vi "Auto.vi"() -> ()   [LabVIEW 2020]
uses:
  Global_Variable/A180648.vi
  Global_Variable/Global.vi
  Libraries/S7/S7.lvlib
  <userlib>/_MGI/1D Array/MGI Running Average/MGI Running Average(DBL[]).vi
panel:
  out "标尺_Event":refnum<user-event>
  in  "STEP":string
  in  "更换坐标":refnum<vi>
  out "试验项_Event":refnum<user-event>
  out "NVH":bool=TRUE
  out "T1+T2":dbl
  out "T2":dbl
  out "T1":dbl
  out "吸收电流":sgl
  out "输出扭矩(大)":sgl
  out "输入扭矩":sgl
  out "力特性逆向去程":bool
  out "力特性正向去程":bool
  out "力特性逆向回程":bool
  out "力特性正向回程":bool
  out "逆向空载正向初始化":bool
  out "锁紧/开启初始化":bool
  out "功能正向初始化":bool
  out "功能逆向初始化":bool
  out "空载逆向初始化":bool
  out "空载正向初始化":bool
  out "当前车速":i32
  out "试验项目":T1(tab)
  out "手柄锁紧力试验":cluster{dbl[], dbl[]}[](graph)
  out "手柄开启力试验":cluster{dbl[], dbl[]}[](graph)
  out "角度调节力试验":cluster{dbl[], dbl[]}[](graph)
  out "管柱保持力试验":cluster{dbl[], dbl[]}[](graph)
  out "锁紧/开启":cluster{dbl[], dbl[]}[](graph)
  out "逆向空载试验":cluster{dbl[], dbl[]}[](graph)
  out "振动2NHV-FFT":cluster{"f0":dbl, "df":dbl, "magnitude":dbl[]}[](graph)
  out "振动1NVH-FFT":cluster{"f0":dbl, "df":dbl, "magnitude":dbl[]}[](graph)
  in  "判定结果":bool[][](array[boolean])=[[TRUE]]
  # "."
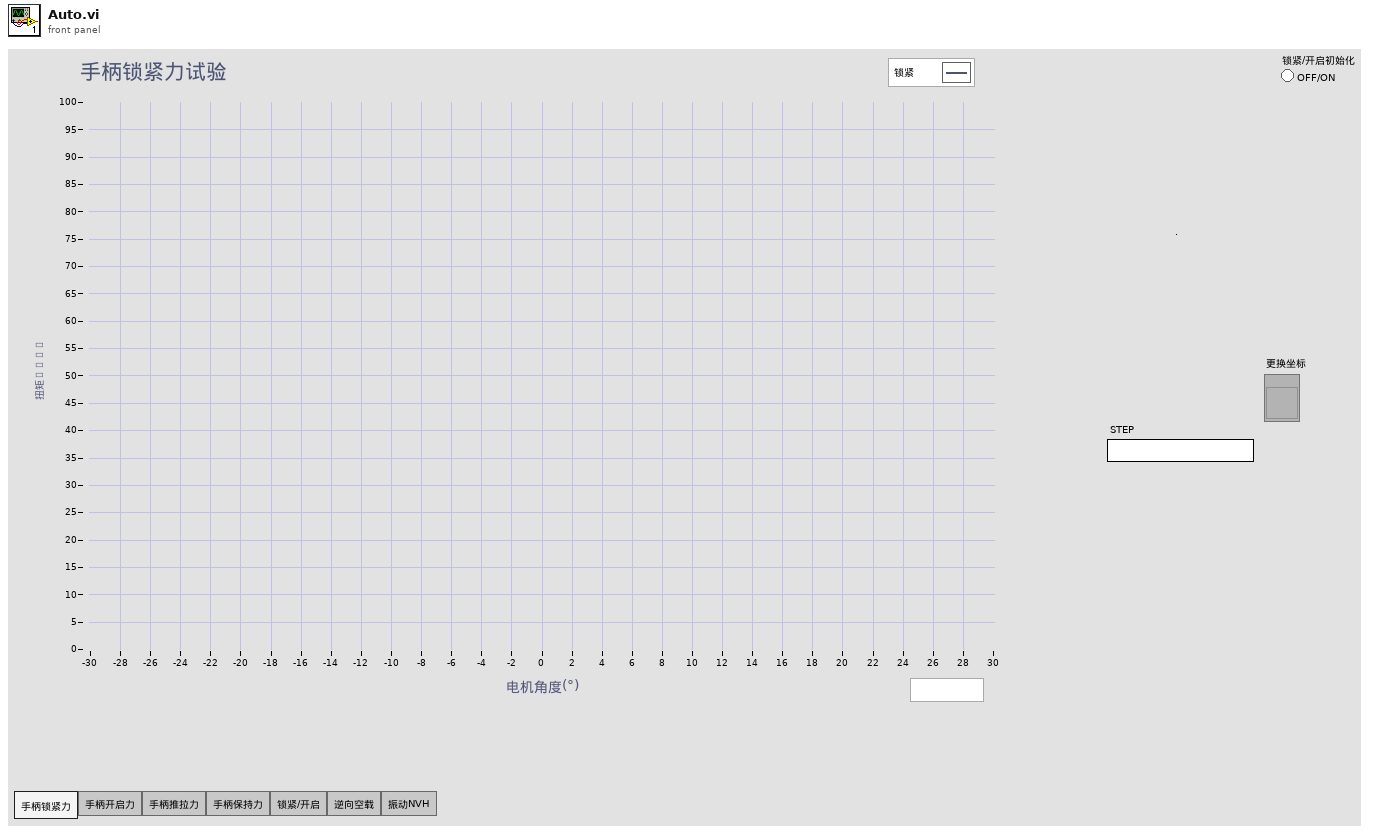
[diagram p1: front panel]
types:
  T1 = enum32{"手柄锁紧力", "手柄开启力", "手柄推拉力", "手柄保持力", "锁紧/开启", "逆向空载", "振动NVH"}
  T2 = enum32{"Invalid", "Standard", "Closed", "Hidden", "Minimized", "Maximized"}
  T3 = enum32{"手柄锁紧力", "手柄开启力", "手柄推拉力", "手柄保持力", "锁紧/开启", "逆向空载", "振动NVH", "完成"}
  T4 = cluster{"输入轴扭矩":dbl, "输出轴扭矩小量程":dbl, "输出轴扭矩大量程":dbl}
  T5 = cluster{"锁紧判断范围":cluster{"单位":string, "下限":dbl, "上限":dbl}}
  T6 = cluster{"开启判断范围":cluster{"单位":string, "下限":dbl, "上限":dbl}}
  T7 = cluster{"推拉力判断范围 ":cluster{"单位":string, "下限":dbl, "上限":dbl}}
  T8 = cluster{"保持力判断范围 ":cluster{"单位":string, "下限":dbl, "上限":dbl}, "保持力监控位移":cluster{"单位":string, "下限":dbl, "上限":dbl}}
  T9 = typedef "lveventtype.ctl" = enum32{"Null", "Timeout", "Annotation Menu Selection", "Annotation Menu Selection?", "App Instance Close", "App Instance Close?", "Autoscale Range Change", "Bookmark Info Change", "Cell Edit", "Cell Edit?", "Cursor Grab", "Cursor Grab?", "Cursor Menu Selection", "Cursor Menu Selection?", "Cursor Move", "Cursor Release", "Data Change", "Direction Change", "Display State Change", "Drag Ended", "Drag Enter", "Drag Leave", "Drag Over", "Drag Source Update", "Drag Starting", "Drag Starting?", "Drop", "Exec State Change", "Key Down", "Key Down?", "Key Repeat", "Key Repeat?", "Key Up", "Listbox Double Click", "Menu Activation?", "Menu Selection (App)", "Menu Selection? (App)", "Menu Selection (User)", "Mouse Down", "Mouse Down?", "Mouse Enter", "Mouse Leave", "Mouse Move", "Mouse Up", "Mouse Wheel", "NI Security User Change (App)", "Pane Size", "Panel Close", "Panel Close?", "Panel Resize", "Plot Attribute Change", "Scale Range Change", "Shortcut Menu Activation?", "Shortcut Menu Selection (App)", "Shortcut Menu Selection? (App)", "Shortcut Menu Selection (User)", "Tree Double Click", "Tree Drag", "Tree Drag?", "Tree Drop", "Tree Drop?", "Tree Item Close", "Tree Item Close?", "Tree Item Open", "Tree Item Open?", "User Event", "Value Change"}
  T10 = typedef "LVPoint32TypeDef.ctl" = cluster{"Horizontal":i32, "Vertical":i32}
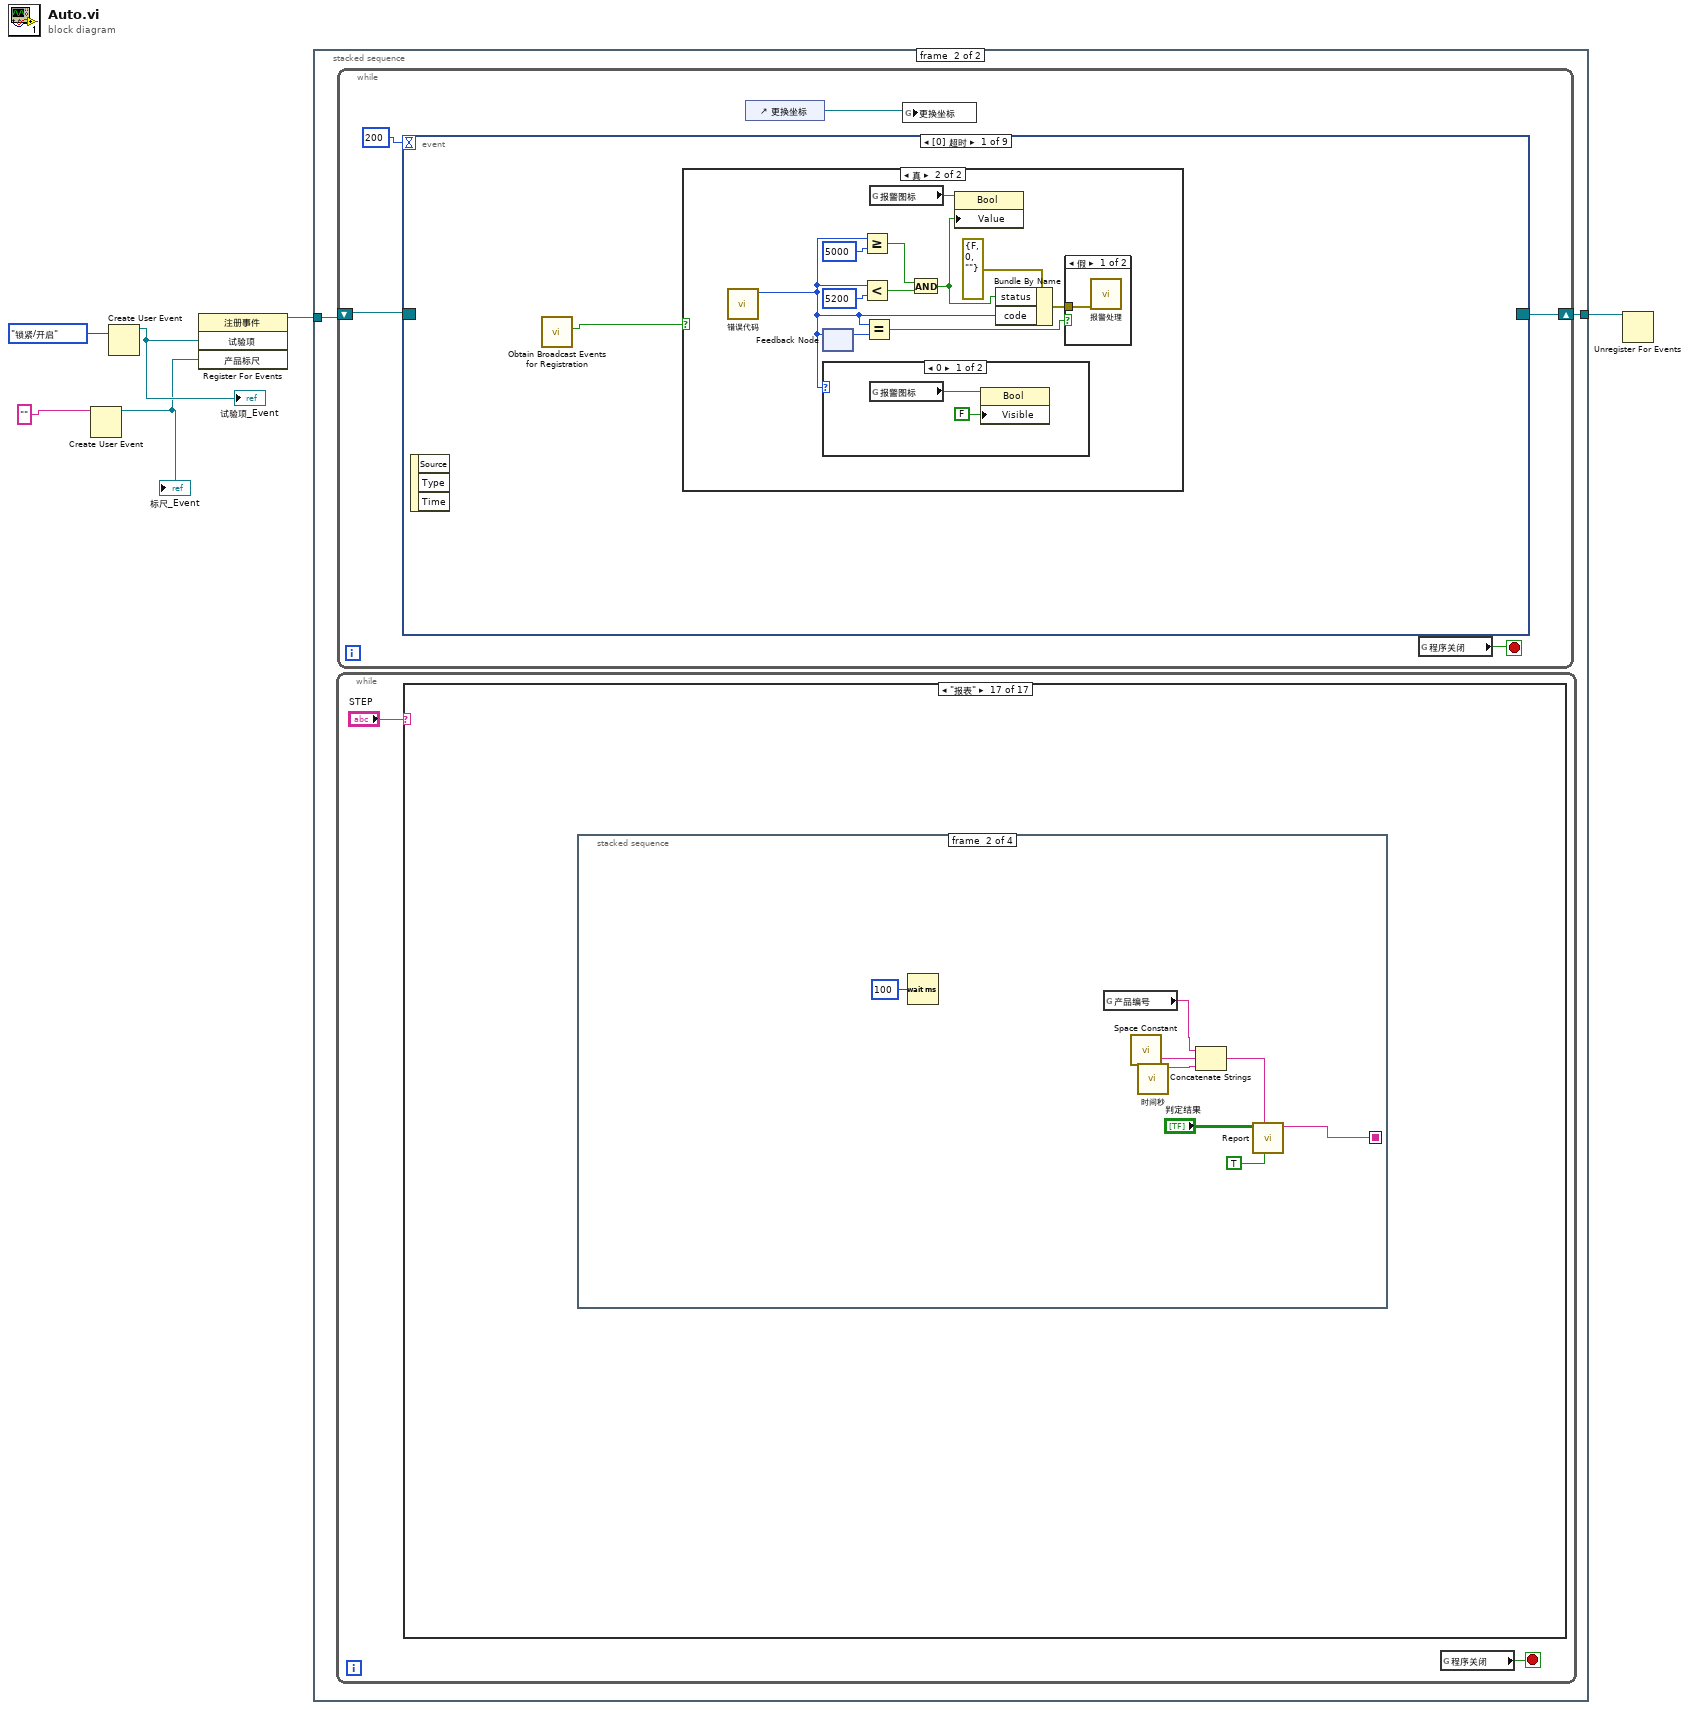
[diagram p0: block diagram]
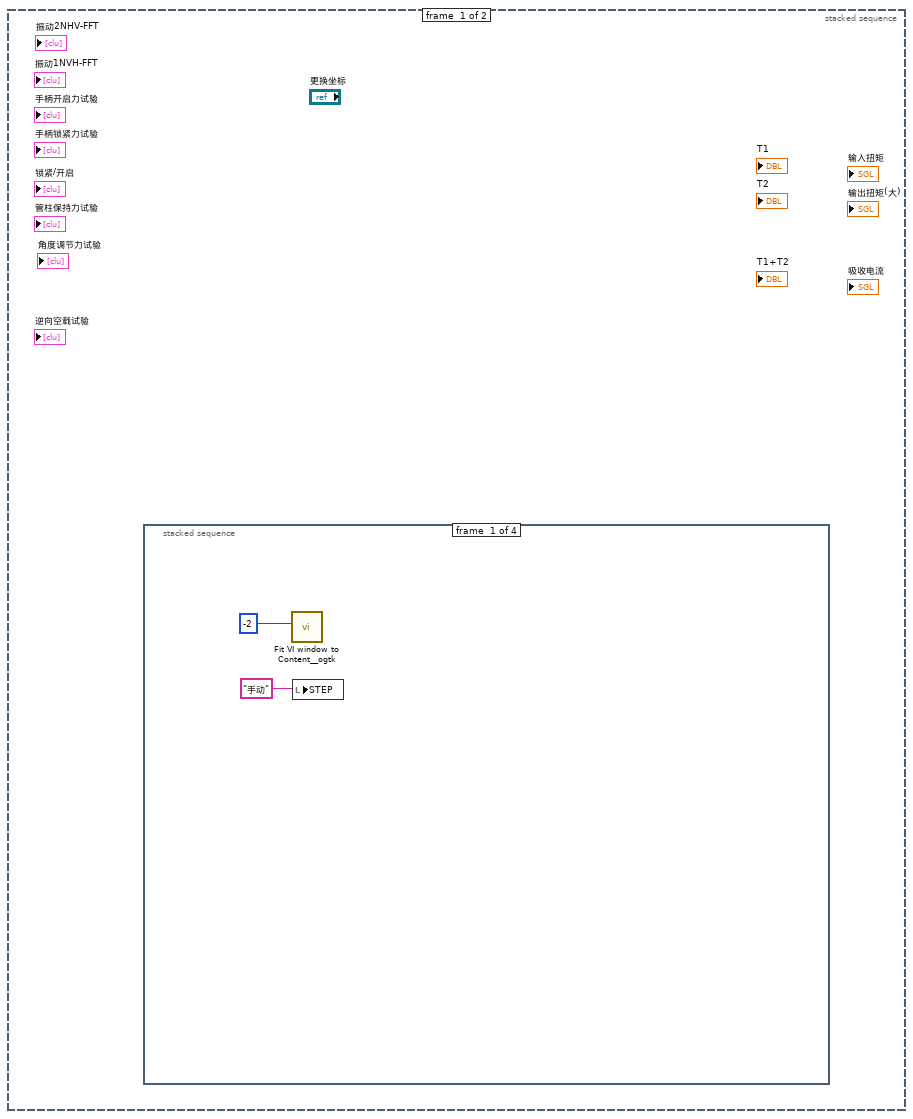
[diagram p2: hidden frame]
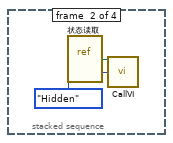
[diagram p3: hidden frame]
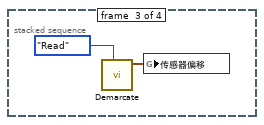
[diagram p4: hidden frame]
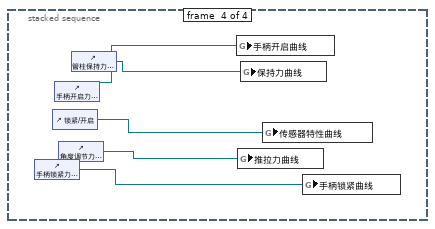
[diagram p5: hidden frame]
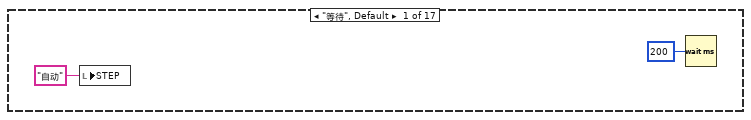
[diagram p6: hidden frame]
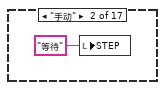
[diagram p7: hidden frame]
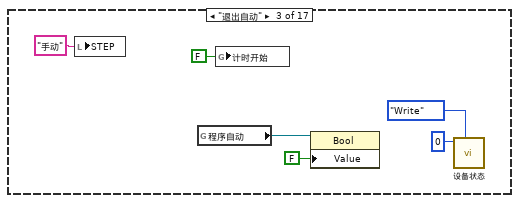
[diagram p8: hidden frame]
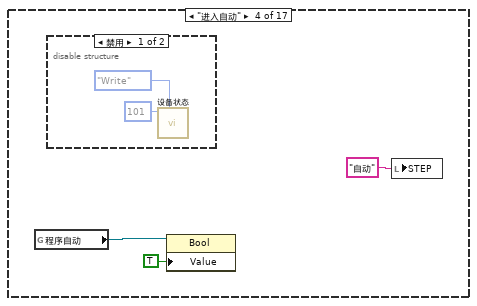
[diagram p9: hidden frame]
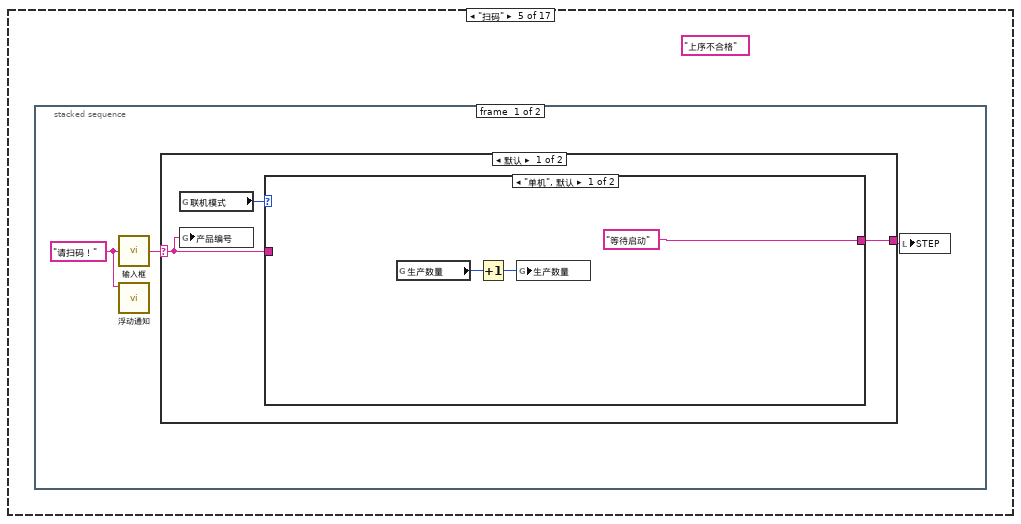
[diagram p11: hidden frame]
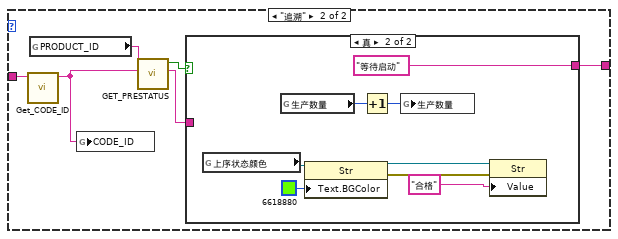
[diagram p12: hidden frame]
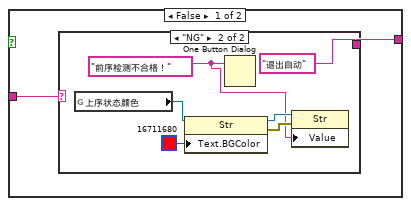
[diagram p13: hidden frame]
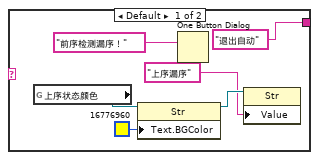
[diagram p14: hidden frame]
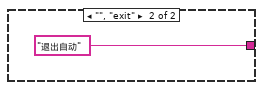
[diagram p15: hidden frame]
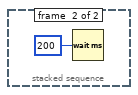
[diagram p16: hidden frame]
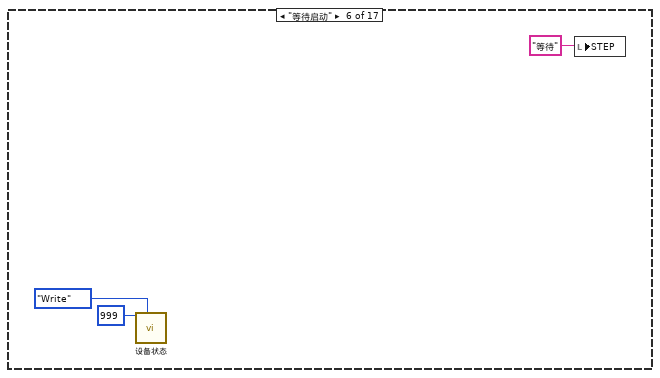
[diagram p17: hidden frame]
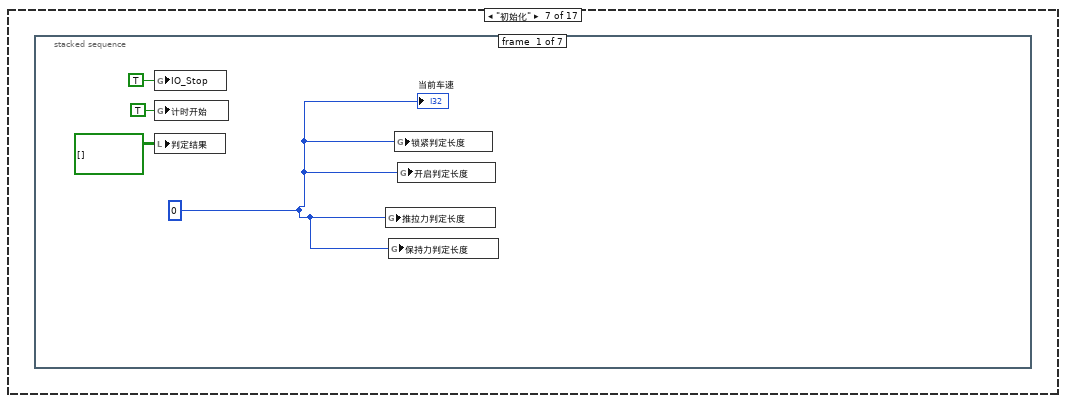
[diagram p18: hidden frame]
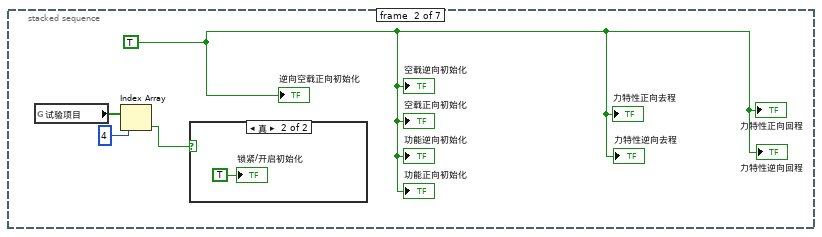
[diagram p19: hidden frame]
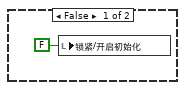
[diagram p20: hidden frame]
diagram:
  n1 = Create User Event(user event datatype="" ("产品标尺")) -> (user event=w2:refnum<user-event>)  [unwired: 1 in, 1 out]
  "标尺_Event" <- w2
  n2 = Create User Event(user event datatype=T1."锁紧/开启" ("试验项")) -> (user event=w3:refnum<user-event>)  [unwired: 1 in, 1 out]
  "试验项_Event" <- w3
  n3 = register-events(w3, w2) -> (reference out=w4:refnum<event-registration>)  [unwired: 2 in, 1 out]
  n4 = stacked-sequence {
    tunnel: [_ w19] -> w6
    tunnel: w4 -> [_ w18]
    frame #0 {
      n5 = stacked-sequence {
        frame #0 {
          n6 = call <userlib>:"Fit VI window to Content__ogtk.vi"("border spacing (2 px)"=-2) -> ()  [unwired: 5 in, 2 out]
          n7 = local write "STEP"("手动" ("STEP")) -> ()
        }
        frame #1 {
          n8 = vi-ref "状态读取.vi"() -> (w10:refnum<vi>)
          n9 = call "CallVI.vi"("VI引用"=w10, "状态"=T2."Hidden") -> ()  [unwired: 12 in, 2 out]
        }
        frame #2 {
          n10 = call "Demarcate.vi"("Mode"=enum16{"Read", "Write"}."Read") -> ("Sensor OUT"=w12:T4)  [unwired: 9 in, 1 out]
          n11 = global write "传感器偏移.vi" "传感器偏移"(w12) -> ()
        }
        frame #3 {
          n12 = control-ref of="手柄锁紧力试验"() -> (w13:refnum<vi>)
          n13 = control-ref of="锁紧/开启"() -> (w15:refnum<vi>)
          n14 = control-ref of="手柄开启力试验"() -> (w14:refnum<vi>)
          n15 = control-ref of="角度调节力试验"() -> (w17:refnum<vi>)
          n16 = control-ref of="管柱保持力试验"() -> (w16:refnum<vi>)
          n17 = global write "A180648.vi" "手柄开启曲线"(w14) -> ()
          n18 = global write "A180648.vi" "推拉力曲线"(w17) -> ()
          n19 = global write "A180648.vi" "保持力曲线"(w16) -> ()
          n20 = global write "A180648.vi" "传感器特性曲线"(w15) -> ()
          n21 = global write "A180648.vi" "手柄锁紧曲线"(w13) -> ()
        }
      }
    }
    frame #1 {
      n22 = while {
        stop <- w21 stop-if-true
        n23 = case shown="\"报表\"" "STEP" {
          frame "等待", Default {
            n24 = local write "STEP"("自动" ("STEP")) -> ()
            n25 = Wait (ms)(milliseconds to wait=u32 200 ("等待时间（毫秒）")) -> ()  [unwired: 1 out]
          }
          frame "手动" {
            n26 = local write "STEP"("等待" ("STEP")) -> ()
          }
          frame "退出自动" {
            n27 = local write "STEP"("手动" ("STEP")) -> ()
            n28 = global read "Global.vi" "程序自动"() -> (w26:refnum<vi>)
            n29 = global write "Global.vi" "计时开始"(FALSE ("计时开始")) -> ()
            n30 = property class="Bool"(reference=w26, "Value"=FALSE) -> ()  [unwired: 1 in, 2 out]
            n31 = call "设备状态.vi"("枚举"=enum16{"Read", "Write"}."Write", "Status_Write"=i16 0) -> ()  [unwired: 9 in, 1 out]
          }
          frame "进入自动" {
            n32 = global read "Global.vi" "程序自动"() -> (w32:refnum<vi>)
            n33 = disable-structure shown="禁用" {
              frame Disabled {
                n34 = call "设备状态.vi"("枚举"=enum16{"Read", "Write"}."Write", "Status_Write"=i16 101) -> ()  [unwired: 9 in, 1 out]
              }
              frame Enabled {
              }
            }
            n35 = property class="Bool"(reference=w32, "Value"=TRUE) -> ()  [unwired: 1 in, 2 out]
            n36 = local write "STEP"("自动" ("STEP")) -> ()
          }
          frame "扫码" {
            (unwired) "上序不合格" ("上序状态")
            n37 = stacked-sequence {
              frame #0 {
                w37 = "请扫码！" ("提示信息")
                n38 = call "输入框.vi"("提示信息"=w37) -> ("条形码输出"=w38:string)
                n39 = call "浮动通知.vi"("通知内容"=w37) -> ()  [unwired: 11 in]
                n40 = case shown="默认" w38 {
                  selector: w38 -> [w40 _]
                  tunnel: [w41 "退出自动" ("State(s) in Front (\"\")")] -> w36
                  frame Default {
                    n41 = global read "Global.vi" "联机模式"() -> (w39:enum16{"单机", "追溯"})
                    n42 = global write "Global.vi" "产品编号"(w40) -> ()
                    n43 = case shown="\"单机\", 默认" w39 {
                      tunnel: ["等待启动" ("State(s) in Front (\"\")") w50] -> w41
                      tunnel: w40 -> [_ w47]
                      frame "单机", Default {
                        n44 = global read "Global.vi" "生产数量"() -> (w42:i32)
                        n45 = Increment(x=w42) -> (x+1=w43:i32)
                        n46 = global write "Global.vi" "生产数量"(w43) -> ()
                      }
                      frame "追溯" {
                        n47 = call "Get_CODE_ID.vi"("CODE_MAIN"=w47) -> ("CODE_ID"=w46:string)  [unwired: 10 in]
                        n48 = global read "追溯Global.vi" "PRODUCT_ID"() -> (w49:string)
                        n49 = global write "追溯Global.vi" "CODE_ID"(w46) -> ()
                        n50 = call "GET_PRESTATUS.vi"("CODE_ID"=w46, "PRODUCT_ID"=w49) -> ("字符串"=w45:string, "OK?"=w48:bool)  [unwired: 8 in]
                        n51 = case shown="真" w48 {
                          tunnel: [w52 "等待启动" ("State(s) in Front (\"\")")] -> w50
                          tunnel: w45 -> [w51 _]
                          frame False {
                            n52 = case shown="\"NG\"" w51 {
                              tunnel: ["退出自动" ("State(s) in Front (\"\")") "退出自动" ("State(s) in Front (\"\")")] -> w52
                              frame Default {
                                n53 = global read "Global.vi" "上序状态颜色"() -> (w58:refnum<vi>)
                                n54 = property class="Str"(reference=w58, "Text.BGColor"=u32 16776960 ("文本.文本颜色:背景色")) -> (reference out=w54:refnum<vi>)  [unwired: 1 in, 1 out]
                                n55 = One Button Dialog(message="前序检测漏序！" ("消息")) -> ()  [unwired: 1 in, 1 out]
                                n56 = property class="Str"(reference=w54, "Value"="上序漏序" ("上序状态")) -> ()  [unwired: 1 in, 2 out]
                              }
                              frame "NG" {
                                w59 = "前序检测不合格！" ("消息")
                                n57 = global read "Global.vi" "上序状态颜色"() -> (w63:refnum<vi>)
                                n58 = property class="Str"(reference=w63, "Text.BGColor"=u32 16711680 ("文本.文本颜色:背景色")) -> (reference out=w61:refnum<vi>, error out=w60:errorcluster)  [unwired: 1 in]
                                n59 = One Button Dialog(message=w59) -> ()  [unwired: 1 in, 1 out]
                                n60 = property class="Str"(reference=w61, error in=w60, "Value"=w59) -> ()  [unwired: 2 out]
                              }
                            }
                          }
                          frame True {
                            n61 = global read "Global.vi" "上序状态颜色"() -> (w69:refnum<vi>)
                            n62 = global read "Global.vi" "生产数量"() -> (w70:i32)
                            n63 = property class="Str"(reference=w69, "Text.BGColor"=u32 6618880 ("文本.文本颜色:背景色")) -> (reference out=w67:refnum<vi>, error out=w66:errorcluster)  [unwired: 1 in]
                            n64 = Increment(x=w70) -> (x+1=w71:i32)
                            n65 = global write "Global.vi" "生产数量"(w71) -> ()
                            n66 = property class="Str"(reference=w67, error in=w66, "Value"="合格" ("上序状态")) -> ()  [unwired: 2 out]
                          }
                        }
                      }
                    }
                  }
                  frame "", "exit" {
                  }
                }
                n67 = local write "STEP"(w36) -> ()
              }
              frame #1 {
                n68 = Wait (ms)(milliseconds to wait=u32 200 ("等待时间（毫秒）")) -> ()  [unwired: 1 out]
              }
            }
          }
          frame "等待启动" {
            n69 = call "设备状态.vi"("枚举"=enum16{"Read", "Write"}."Write", "Status_Write"=i16 999 ("设备状态")) -> ()  [unwired: 9 in, 1 out]
            n70 = local write "STEP"("等待" ("STEP")) -> ()
          }
          frame "初始化" {
            n71 = stacked-sequence {
              frame #0 {
                w78 = 0 ("当前车速")
                n72 = global write "Global.vi" "IO_Stop"(TRUE ("IO_Stop")) -> ()
                n73 = global write "Global.vi" "计时开始"(TRUE ("计时开始")) -> ()
                n74 = local write "判定结果"(bool[][] [] ("判定结果")) -> ()
                n75 = global write "判定参数.vi" "推拉力判定长度"(w78) -> ()
                n76 = global write "判定参数.vi" "保持力判定长度"(w78) -> ()
                n77 = global write "判定参数.vi" "锁紧判定长度"(w78) -> ()
                n78 = global write "判定参数.vi" "开启判定长度"(w78) -> ()
                "当前车速" <- w78
              }
              frame #1 {
                w85 = TRUE
                n79 = global read "Global.vi" "试验项目"() -> (w84:bool[])
                n80 = Index Array(array=w84, index=4 ("索引")) -> (element=w82:bool)
                n81 = case shown="真" w82 {
                  frame False {
                    n82 = local write "锁紧/开启初始化"(FALSE ("锁紧/开启初始化")) -> ()
                  }
                  frame True {
                    "锁紧/开启初始化" <- TRUE ("锁紧/开启初始化")
                  }
                }
                "逆向空载正向初始化" <- w85
                "空载正向初始化" <- w85
                "空载逆向初始化" <- w85
                "功能正向初始化" <- w85
                "功能逆向初始化" <- w85
                "力特性逆向去程" <- w85
                "力特性正向去程" <- w85
                "力特性逆向回程" <- w85
                "力特性正向回程" <- w85
              }
              frame #2 {
                n83 = for {
                  N: 24 -> [_]
                  tunnel: [cluster{dbl[], dbl[]} {[], []}] -> w89 mode=indexing
                  tunnel: [cluster{"f0":dbl, "df":dbl, "magnitude":dbl[]} {"f0"=0.0, "df"=0.0, "magnitude"=[]} ("power spectrum [dB EU]")] -> w88 mode=indexing
                }
                n84 = local write "角度调节力试验"(w89) -> ()
                n85 = local write "管柱保持力试验"(w89) -> ()
                n86 = local write "手柄锁紧力试验"(w89) -> ()
                n87 = local write "手柄开启力试验"(w89) -> ()
                n88 = local write "逆向空载试验"(w89) -> ()
                n89 = local write "锁紧/开启"(w89) -> ()
                n90 = local write "振动2NHV-FFT"(w88) -> ()
                n91 = local write "振动1NVH-FFT"(w88) -> ()
              }
              frame #3 {
                w94 = -2
                n92 = Bundle(w94, w94) -> (w93:cluster{i32, i32})  [unwired: 1 in]
                n93 = global read "Global.vi" "Result"() -> (w96:refnum<vi>)
                n94 = property class="Tbl"(reference=w96, "Active Cell"=w93, "Cell BG Color"=u32 16777216 ("活动单元格:单元格背景色")) -> ()  [unwired: 1 in, 2 out]
                n95 = property class="Tbl"(reference=w96, "Value"=string[][] []) -> (reference out=w99:refnum<vi>, error out=w100:errorcluster)  [unwired: 1 in]
                n96 = property class="Tbl"(reference=w99, error in=w100, "Row Headers[]"=string[] [] ("列首字符串[]")) -> ()  [unwired: 2 out]
              }
              frame #4 {
                n97 = global read "A180648.vi" "LED-手柄锁紧力"() -> (w102:refnum<vi>)
                n98 = global read "A180648.vi" "LED-手柄开启力"() -> (w103:refnum<vi>)
                n99 = global read "A180648.vi" "LED-推拉力"() -> (w105:refnum<vi>)
                n100 = global read "A180648.vi" "LED-保持力"() -> (w101:refnum<vi>)
                n101 = Build Array(w102, w103, w105, w101) -> (w104:refnum<vi>[])
                n102 = for {
                  tunnel: w104 -> [w106] mode=indexing
                  n103 = property class="Bool"(reference=w106, "Colors [4]"=cluster{u32, u32}[] [{12369084, 12369084}] ("颜色[4]")) -> ()  [unwired: 1 in, 2 out]
                }
              }
              frame #5 {
                n104 = global read "Global.vi" "启用CAN"() -> (w108:bool)
                n105 = case shown="真" w108 {
                  frame False {
                  }
                  frame True {
                    n106 = call "循环发送CAN.vi"() -> ()  [unwired: 11 in, 1 out]
                  }
                }
              }
              frame #6 {
                w111 = 1 ("维数大小")
                n107 = local write "STEP"("试验项" ("STEP")) -> ()
                n108 = global write "Global.vi" "STOP_NVH"(FALSE ("STOP_NVH")) -> ()
                n109 = global write "A180648.vi" "当前检测项"(T3."手柄锁紧力" ("值(信号)")) -> ()
                n110 = Initialize Array(" " ("字符串"), w111, w111, w111) -> (w113:string[][][])
                n111 = global write "A180648.vi" "检测结果"(w113) -> ()
              }
            }
          }
          frame "试验项" {
            n112 = global read "A180648.vi" "当前检测项"() -> (w115:T3)
            n113 = case shown="\"手柄锁紧力\", 默认" w115 {
              selector: w115 -> [w117 _]
              tunnel: [w120 "报表" ("STEP")] -> w116
              frame "手柄锁紧力", Default {
                n114 = global read "Global.vi" "试验项目"() -> (w118:bool[])
                n115 = Index Array(array=w118, index=w117) -> (element=w119:bool)
                n116 = case shown="假" w119 {
                  tunnel: ["试验项" ("字符串") w127] -> w120
                  tunnel: w117 -> [_ w128]
                  frame False {
                    n117 = global read "A180648.vi" "当前检测项"() -> (w125:T3)
                    n118 = Increment(x=w125) -> (x+1=w124:T3)
                    n119 = global write "A180648.vi" "当前检测项"(w124) -> ()
                    n120 = local read "判定结果"() -> (w121:bool[][])
                    n121 = Build Array (concatenate)(w121, bool[] [FALSE] ("判定结果")) -> (w122:bool[][])
                    n122 = local write "判定结果"(w122) -> ()
                  }
                  frame True {
                    n123 = case shown="\"手柄保持力\"" w128 {
                      tunnel: ["手柄锁紧力" ("STEP") "手柄开启力" ("STEP") "手柄推拉力" ("STEP") "手柄保持力" ("STEP") "套输入轴花键" ("STEP") w155 "退输入轴花键" ("STEP")] -> w127
                      frame "手柄锁紧力", Default {
                        n124 = call "浮动通知.vi"("通知内容"="手柄锁紧力试验") -> ()  [unwired: 11 in]
                        n125 = property on="试验项目" class="TabCtl (严格)"("Val(Sgnl)"=T1."手柄锁紧力" ("值(信号)")) -> ()  [unwired: 2 in, 2 out]
                      }
                      frame "手柄开启力" {
                        n126 = call "浮动通知.vi"("通知内容"="手柄开启力试验") -> ()  [unwired: 11 in]
                        n127 = property on="试验项目" class="TabCtl (严格)"("Val(Sgnl)"=T1."手柄开启力" ("值(信号)")) -> ()  [unwired: 2 in, 2 out]
                      }
                      frame "手柄推拉力" {
                        n128 = call "浮动通知.vi"("通知内容"="角度调节力试验") -> ()  [unwired: 11 in]
                        n129 = property on="试验项目" class="TabCtl (严格)"("Val(Sgnl)"=T1."手柄推拉力" ("值(信号)")) -> ()  [unwired: 2 in, 2 out]
                      }
                      frame "手柄保持力" {
                        n130 = call "浮动通知.vi"("通知内容"="管柱保持力试验") -> ()  [unwired: 11 in]
                        n131 = property on="试验项目" class="TabCtl (严格)"("Val(Sgnl)"=T1."手柄保持力" ("值(信号)")) -> ()  [unwired: 2 in, 2 out]
                      }
                      frame "完成" {
                        n132 = for {
                          tunnel: sgl[] [1.0, 15.0] ("力特性参数") -> [w144] mode=indexing
                          i -> [w147]
                          w152 = u16 2 items=["byte", "word", "Dword"] ("数据类型")
                          w154 = u8 132 items=["I/O (P)"=128, "Input (I)"=129, "Output (Q)"=130, "Bit Memory (M)"=131, "Data (DB)"=132, "Instance Data (DI)"=133, "Local Data (L)"=134, "Predecessor Local Data (VL)"=135] ("寄存器类型")
                          n133 = Type Cast(type=u32 0 ("写入地址"), x=w144) -> (*(type *) &x=w150:u32)
                          n134 = Multiply(x=w147, y=4) -> (x*y=w148:i32)
                          n135 = Add(x=u32 152 ("写入地址"), y=w148) -> (x+y=w145:u32)
                          n136 = call "Write_Data.vi"("DB #"=u16 7, "寄存器类型"=w154, "写入数据"=w150, "数据类型"=w152, "写入地址"=w145) -> ()  [unwired: 4 in, 3 out]
                        }
                        n137 = call "浮动通知.vi"("通知内容"="传感器特性试验") -> ()  [unwired: 11 in]
                      }
                      frame "振动NVH" {
                        n138 = call "浮动通知.vi"("通知内容"="振动NVH试验") -> ()  [unwired: 11 in]
                        n139 = local read "NVH"() -> (w158:bool)
                        n140 = Select(t="判定" ("STEP"), s=w158, f="退输入轴花键" ("STEP")) -> (s? t:f=w155:string)
                      }
                      frame "逆向空载" {
                        n141 = call "浮动通知.vi"("通知内容"="逆向空载试验") -> ()  [unwired: 11 in]
                      }
                    }
                  }
                }
              }
              frame "完成" {
                n142 = call "浮动通知.vi"("通知内容"="试验完成") -> ()  [unwired: 11 in]
                n143 = call "设备状态.vi"("枚举"=enum16{"Read", "Write"}."Write", "Status_Write"=i16 100 ("设备状态")) -> ()  [unwired: 9 in, 1 out]
                n144 = Wait (ms)(milliseconds to wait=u32 100 ("等待时间（毫秒）")) -> ()  [unwired: 1 out]
              }
            }
            n145 = local write "STEP"(w116) -> ()
          }
          frame "判定" {
            n146 = stacked-sequence {
              frame #0 {
                n147 = global read "A180648.vi" "当前检测项"() -> (w167:T3)
                n148 = case shown="\"手柄推拉力\"" w167 {
                  frame "完成", Default {
                  }
                  frame "手柄锁紧力" {
                    n149 = global read "判定参数.vi" "锁紧判定参数"() -> (w179:T5)
                    n150 = local read "手柄锁紧力试验"() -> (w180:cluster{dbl[], dbl[]}[])
                    n151 = global read "A180648.vi" "LED-手柄锁紧力"() -> (w174:refnum<vi>)
                    n152 = global read "Global.vi" "Result"() -> (w178:refnum<vi>)
                    n153 = call "锁紧试验判定.vi"("Result"=w178, "判定参数"=w179, "XY曲线"=w180) -> ("判定项长度"=w169:i32, "OK？"=w168:bool)  [unwired: 7 in]
                    n154 = Select(t=cluster{u32, u32}[] [{6618880, 6618880}, {6618880, 6618880}, {6618880, 6618880}, {6618880, 6618880}] ("颜色[4]"), s=w168, f=cluster{u32, u32}[] [{16711680, 16711680}, {16711680, 16711680}, {16711680, 16711680}, {16711680, 16711680}] ("颜色[4]")) -> (s? t:f=w175:cluster{u32, u32}[])
                    n155 = property class="Bool"(reference=w174, "Colors [4]"=w175) -> ()  [unwired: 1 in, 2 out]
                    n156 = local read "判定结果"() -> (w170:bool[][])
                    n157 = Build Array(TRUE, w168) -> (w173:bool[])
                    n158 = global write "判定参数.vi" "锁紧判定长度"(w169) -> ()
                    n159 = Build Array (concatenate)(w170, w173) -> (w171:bool[][])
                    n160 = case shown="假" w168 {
                      frame False {
                        n161 = call "合格状态.vi"("枚举"=enum16{"Read", "Write"}."Write", "起始地址"=u32 180, "Status_Write"=i16 2) -> ()  [unwired: 8 in, 1 out]
                      }
                      frame True {
                        n162 = call "合格状态.vi"("枚举"=enum16{"Read", "Write"}."Write", "起始地址"=u32 180, "Status_Write"=i16 1) -> ()  [unwired: 8 in, 1 out]
                      }
                    }
                    n163 = local write "判定结果"(w171) -> ()
                  }
                  frame "手柄开启力" {
                    n164 = local read "手柄开启力试验"() -> (w200:cluster{dbl[], dbl[]}[])
                    n165 = global read "A180648.vi" "LED-手柄开启力"() -> (w194:refnum<vi>)
                    n166 = global read "判定参数.vi" "开启判定参数"() -> (w199:T6)
                    n167 = global read "Global.vi" "Result"() -> (w198:refnum<vi>)
                    n168 = call "开启试验判定.vi"("Result"=w198, "判定参数"=w199, "XY曲线"=w200) -> ("判定项长度"=w189:i32, "OK？"=w187:bool)  [unwired: 7 in]
                    n169 = Select(t=cluster{u32, u32}[] [{6618880, 6618880}, {6618880, 6618880}, {6618880, 6618880}, {6618880, 6618880}] ("颜色[4]"), s=w187, f=cluster{u32, u32}[] [{16711680, 16711680}, {16711680, 16711680}, {16711680, 16711680}, {16711680, 16711680}] ("颜色[4]")) -> (s? t:f=w195:cluster{u32, u32}[])
                    n170 = property class="Bool"(reference=w194, "Colors [4]"=w195) -> ()  [unwired: 1 in, 2 out]
                    n171 = local read "判定结果"() -> (w190:bool[][])
                    n172 = global write "判定参数.vi" "开启判定长度"(w189) -> ()
                    n173 = Build Array(TRUE, w187) -> (w193:bool[])
                    n174 = Build Array (concatenate)(w190, w193) -> (w191:bool[][])
                    n175 = case shown="假" w187 {
                      frame False {
                        n176 = call "合格状态.vi"("枚举"=enum16{"Read", "Write"}."Write", "起始地址"=u32 76, "Status_Write"=i16 2) -> ()  [unwired: 8 in, 1 out]
                      }
                      frame True {
                        n177 = call "合格状态.vi"("枚举"=enum16{"Read", "Write"}."Write", "起始地址"=u32 76, "Status_Write"=i16 1) -> ()  [unwired: 8 in, 1 out]
                      }
                    }
                    n178 = local write "判定结果"(w191) -> ()
                    "NVH" <- TRUE
                  }
                  frame "手柄推拉力" {
                    n179 = global read "判定参数.vi" "推拉力判定参数"() -> (w210:T7)
                    n180 = local read "角度调节力试验"() -> (w219:cluster{dbl[], dbl[]}[])
                    n181 = global read "A180648.vi" "LED-推拉力"() -> (w217:refnum<vi>)
                    n182 = global read "Global.vi" "Result"() -> (w208:refnum<vi>)
                    n183 = call "推拉力判定.vi"("Result"=w208, "判定参数"=w210, "XY曲线"=w219) -> ("判定项长度"=w209:i32, "OK？"=w207:bool)  [unwired: 7 in]
                    n184 = Select(t=cluster{u32, u32}[] [{6618880, 6618880}, {6618880, 6618880}, {6618880, 6618880}, {6618880, 6618880}] ("颜色[4]"), s=w207, f=cluster{u32, u32}[] [{16711680, 16711680}, {16711680, 16711680}, {16711680, 16711680}, {16711680, 16711680}] ("颜色[4]")) -> (s? t:f=w218:cluster{u32, u32}[])
                    n185 = property class="Bool"(reference=w217, "Colors [4]"=w218) -> ()  [unwired: 1 in, 2 out]
                    n186 = local read "判定结果"() -> (w211:bool[][])
                    n187 = global write "判定参数.vi" "推拉力判定长度"(w209) -> ()
                    n188 = case shown="真" w207 {
                      frame False {
                        n189 = call "合格状态.vi"("枚举"=enum16{"Read", "Write"}."Write", "起始地址"=u32 96, "Status_Write"=i16 2) -> ()  [unwired: 8 in, 1 out]
                      }
                      frame True {
                        n190 = call "合格状态.vi"("枚举"=enum16{"Read", "Write"}."Write", "起始地址"=u32 96, "Status_Write"=i16 1) -> ()  [unwired: 8 in, 1 out]
                      }
                    }
                    n191 = Build Array(TRUE, w207) -> (w214:bool[])
                    n192 = Build Array (concatenate)(w211, w214) -> (w212:bool[][])
                    n193 = local write "判定结果"(w212) -> ()
                  }
                  frame "手柄保持力" {
                    n194 = local read "管柱保持力试验"() -> (w242:cluster{dbl[], dbl[]}[])
                    n195 = global read "判定参数.vi" "保持力判定参数"() -> (w236:T8)
                    n196 = global read "判定参数.vi" "最大拉力"() -> (w227:dbl)
                    n197 = global read "判定参数.vi" "最大拉力"() -> (w226:dbl)
                    n198 = global read "判定参数.vi" "最小位移"() -> (w230:dbl)
                    n199 = global read "判定参数.vi" "最大位移"() -> (w229:dbl)
                    n200 = global read "A180648.vi" "LED-保持力"() -> (w240:refnum<vi>)
                    n201 = global read "Global.vi" "Result"() -> (w231:refnum<vi>)
                    n202 = call "保持力判定.vi"("最大力"=w227, "最小力"=w226, "Result"=w231, "最大位移"=w229, "最小位移"=w230, "判定参数"=w236, "XY曲线"=w242) -> ("判定项长度"=w232:i32, "OK？"=w228:bool)  [unwired: 3 in]
                    n203 = Select(t=cluster{u32, u32}[] [{6618880, 6618880}, {6618880, 6618880}, {6618880, 6618880}, {6618880, 6618880}] ("颜色[4]"), s=w228, f=cluster{u32, u32}[] [{16711680, 16711680}, {16711680, 16711680}, {16711680, 16711680}, {16711680, 16711680}] ("颜色[4]")) -> (s? t:f=w241:cluster{u32, u32}[])
                    n204 = property class="Bool"(reference=w240, "Colors [4]"=w241) -> ()  [unwired: 1 in, 2 out]
                    n205 = local read "判定结果"() -> (w237:bool[][])
                    n206 = case shown="真" w228 {
                      frame False {
                        n207 = call "合格状态.vi"("枚举"=enum16{"Read", "Write"}."Write", "起始地址"=u32 116, "Status_Write"=i16 2) -> ()  [unwired: 8 in, 1 out]
                      }
                      frame True {
                        n208 = call "合格状态.vi"("枚举"=enum16{"Read", "Write"}."Write", "起始地址"=u32 116, "Status_Write"=i16 1) -> ()  [unwired: 8 in, 1 out]
                      }
                    }
                    n209 = global write "判定参数.vi" "保持力判定长度"(w232) -> ()
                    n210 = Build Array(TRUE, w228) -> (w239:bool[])
                    n211 = Build Array (concatenate)(w237, w239) -> (w238:bool[][])
                    n212 = local write "判定结果"(w238) -> ()
                  }
                }
              }
              frame #1 {
                n213 = call "合格状态.vi"("枚举"=enum16{"Read", "Write"}."Read", "起始地址"=u32 76) -> ("Status_Read"=w249:i16)  [unwired: 9 in]
                n214 = case shown="2" w249 {
                  frame 2 {
                    n215 = call "合格状态.vi"("枚举"=enum16{"Read", "Write"}."Read", "起始地址"=u32 86) -> ("Status_Read"=w259:i16)  [unwired: 9 in]
                    n216 = call "合格状态.vi"("枚举"=enum16{"Read", "Write"}."Read", "起始地址"=u32 106) -> ("Status_Read"=w256:i16)  [unwired: 9 in]
                    n217 = call "合格状态.vi"("枚举"=enum16{"Read", "Write"}."Read", "起始地址"=u32 58) -> ("Status_Read"=w255:i16)  [unwired: 9 in]
                    n218 = Greater Or Equal?(x=w256, y=w255) -> (x >= y?=w253:bool)
                    n219 = Greater Or Equal?(x=w259, y=w255) -> (x >= y?=w254:bool)
                    n220 = Or(x=w254, y=w253) -> (x .or. y?=w252:bool)
                    n221 = case shown="真" w252 {
                      frame False {
                        n222 = local write "STEP"("等待" ("STEP")) -> ()
                        n223 = call "设备状态.vi"("枚举"=enum16{"Read", "Write"}."Write", "Status_Write"=i16 52) -> ()  [unwired: 9 in, 1 out]
                      }
                      frame True {
                        n224 = local write "STEP"("试验项" ("STEP")) -> ()
                        n225 = global write "A180648.vi" "当前检测项"(T3."完成" ("当前检测项")) -> ()
                      }
                    }
                  }
                  frame 1 {
                    n226 = call "合格状态.vi"("枚举"=enum16{"Read", "Write"}."Read", "起始地址"=u32 180) -> ("Status_Read"=w269:i16)  [unwired: 9 in]
                    n227 = case shown="1" w269 {
                      frame 0, Default {
                      }
                      frame 1 {
                        n228 = global read "A180648.vi" "当前检测项"() -> (w274:T3)
                        n229 = local write "STEP"("试验项" ("STEP")) -> ()
                        n230 = Increment(x=w274) -> (x+1=w273:T3)
                        n231 = global write "A180648.vi" "当前检测项"(w273) -> ()
                      }
                      frame 2 {
                        n232 = call "合格状态.vi"("枚举"=enum16{"Read", "Write"}."Read", "起始地址"=u32 86) -> ("Status_Read"=w286:i16)  [unwired: 9 in]
                        n233 = call "合格状态.vi"("枚举"=enum16{"Read", "Write"}."Read", "起始地址"=u32 106) -> ("Status_Read"=w285:i16)  [unwired: 9 in]
                        n234 = call "合格状态.vi"("枚举"=enum16{"Read", "Write"}."Read", "起始地址"=u32 58) -> ("Status_Read"=w284:i16)  [unwired: 9 in]
                        n235 = Greater Or Equal?(x=w285, y=w284) -> (x >= y?=w282:bool)
                        n236 = Greater Or Equal?(x=w286, y=w284) -> (x >= y?=w283:bool)
                        n237 = Or(x=w283, y=w282) -> (x .or. y?=w281:bool)
                        n238 = case shown="假" w281 {
                          frame False {
                            n239 = local write "STEP"("等待" ("STEP")) -> ()
                            n240 = call "设备状态.vi"("枚举"=enum16{"Read", "Write"}."Write", "Status_Write"=i16 52) -> ()  [unwired: 9 in, 1 out]
                          }
                          frame True {
                            n241 = local write "STEP"("试验项" ("STEP")) -> ()
                            n242 = global write "A180648.vi" "当前检测项"(T3."完成" ("当前检测项")) -> ()
                          }
                        }
                      }
                    }
                  }
                  frame 0, Default {
                    n243 = global read "A180648.vi" "当前检测项"() -> (w294:T3)
                    n244 = local write "STEP"("试验项" ("STEP")) -> ()
                    n245 = Increment(x=w294) -> (x+1=w293:T3)
                    n246 = global write "A180648.vi" "当前检测项"(w293) -> ()
                  }
                }
              }
            }
          }
          frame "手柄锁紧力" {
            n247 = disable-structure shown="禁用" {
              frame Disabled {
                n248 = call "设备状态.vi"() -> ("Status_Read"=w298:i16)  [unwired: 11 in]
                n249 = case shown="0, 默认" w298 {
                  frame 0, Default {
                  }
                  frame 103 {
                    n250 = global read "A180648.vi" "当前检测项"() -> (w300:T3)
                    n251 = case shown="\"手柄开启力\"" w300 {
                      tunnel: ["退输出轴花键" ("STEP") "套输出轴花键" ("STEP") "套输出轴花键" ("STEP") "套输出轴花键" ("STEP") "套输出轴花键" ("STEP")] -> w299
                      frame "手柄锁紧力", Default {
                      }
                      frame "手柄开启力" {
                      }
                      frame "手柄推拉力" {
                      }
                      frame "完成" {
                      }
                      frame "手柄保持力" {
                      }
                    }
                    n252 = local write "STEP"(w299) -> ()
                  }
                  frame 1024 {
                    n253 = local write "STEP"("退出自动" ("STEP")) -> ()
                  }
                }
              }
              frame Enabled {
              }
            }
            n254 = local write "STEP"("等待" ("STEP")) -> ()
            n255 = call "设备状态.vi"("枚举"=enum16{"Read", "Write"}."Write", "Status_Write"=i16 40 ("设备状态")) -> ()  [unwired: 9 in, 1 out]
          }
          frame "手柄开启力" {
            n256 = disable-structure shown="禁用" {
              frame Disabled {
                n257 = call "设备状态.vi"() -> ("Status_Read"=w310:i16)  [unwired: 11 in]
                n258 = case shown="105" w310 {
                  frame 0, Default {
                    n259 = call "设备状态.vi"("枚举"=enum16{"Read", "Write"}."Write", "Status_Write"=i16 104 ("设备状态")) -> ()  [unwired: 9 in, 1 out]
                  }
                  frame 105 {
                    n260 = global read "A180648.vi" "当前检测项"() -> (w314:T3)
                    n261 = case shown="\"完成\"" w314 {
                      tunnel: ["自动" ("STEP") "退输出轴花键" ("STEP") "套输出轴花键" ("STEP") "退输出轴花键" ("STEP")] -> w313
                      frame Default {
                      }
                      frame "振动NVH" {
                      }
                      frame "逆向空载" {
                      }
                      frame "完成" {
                      }
                    }
                    n262 = local write "STEP"(w313) -> ()
                  }
                  frame 1024 {
                    n263 = local write "STEP"("退出自动" ("STEP")) -> ()
                  }
                }
              }
              frame Enabled {
              }
            }
            n264 = local write "STEP"("等待" ("STEP")) -> ()
            n265 = call "设备状态.vi"("枚举"=enum16{"Read", "Write"}."Write", "Status_Write"=i16 50 ("设备状态")) -> ()  [unwired: 9 in, 1 out]
          }
          frame "手柄推拉力" {
            n266 = disable-structure shown="禁用" {
              frame Disabled {
                n267 = call "设备状态.vi"() -> ("Status_Read"=w323:i16)  [unwired: 11 in]
                n268 = case shown="107" w323 {
                  frame 0, Default {
                    n269 = call "设备状态.vi"("枚举"=enum16{"Read", "Write"}."Write", "Status_Write"=i16 106 ("设备状态")) -> ()  [unwired: 9 in, 1 out]
                  }
                  frame 107 {
                    n270 = local write "STEP"("设置输出轴模式" ("STEP")) -> ()
                  }
                  frame 1024 {
                    n271 = local write "STEP"("退出自动" ("STEP")) -> ()
                  }
                }
              }
              frame Enabled {
              }
            }
            n272 = local write "STEP"("等待" ("STEP")) -> ()
            n273 = call "设备状态.vi"("枚举"=enum16{"Read", "Write"}."Write", "Status_Write"=i16 60 ("设备状态")) -> ()  [unwired: 9 in, 1 out]
          }
          frame "手柄保持力" {
            n274 = disable-structure shown="禁用" {
              frame Disabled {
                n275 = call "设备状态.vi"() -> ("Status_Read"=w331:i16)  [unwired: 11 in]
                n276 = case shown="109" w331 {
                  frame 0, Default {
                    n277 = call "设备状态.vi"("枚举"=enum16{"Read", "Write"}."Write", "Status_Write"=i16 108 ("设备状态")) -> ()  [unwired: 9 in, 1 out]
                  }
                  frame 109 {
                    n278 = global read "A180648.vi" "当前检测项"() -> (w334:T3)
                    n279 = case shown="默认" w334 {
                      tunnel: ["自动" ("STEP") "自动" ("STEP") "报表" ("STEP") "自动" ("STEP")] -> w335
                      frame Default {
                      }
                      frame "振动NVH" {
                        n280 = call "设备状态.vi"("枚举"=enum16{"Read", "Write"}."Write", "Status_Write"=i16 142 ("设备状态")) -> ()  [unwired: 9 in, 1 out]
                      }
                      frame "完成" {
                        n281 = call "浮动通知.vi"("通知内容"="检测完成！" ("Status")) -> ()  [unwired: 11 in]
                        n282 = call "设备状态.vi"("枚举"=enum16{"Read", "Write"}."Write", "Status_Write"=i16 160) -> ()  [unwired: 9 in, 1 out]
                      }
                      frame "手柄锁紧力" {
                        n283 = call "设备状态.vi"("枚举"=enum16{"Read", "Write"}."Write", "Status_Write"=i16 112) -> ()  [unwired: 9 in, 1 out]
                      }
                    }
                    n284 = local write "STEP"(w335) -> ()
                  }
                  frame 110 {
                    n285 = local write "STEP"("退出自动" ("STEP")) -> ()
                  }
                }
              }
              frame Enabled {
              }
            }
            n286 = local write "STEP"("等待" ("STEP")) -> ()
            n287 = call "设备状态.vi"("枚举"=enum16{"Read", "Write"}."Write", "Status_Write"=i16 70 ("设备状态")) -> ()  [unwired: 9 in, 1 out]
          }
          frame "设置输出轴模式" {
            n288 = global read "A180648.vi" "当前检测项"() -> (w349:T3)
            n289 = case shown="\"手柄开启力\"" w349 {
              tunnel: ["自动" ("STEP") "自动" ("STEP") "自动" ("STEP") "自动" ("STEP") "自动" ("STEP") "自动" ("STEP")] -> w348
              frame Default {
              }
              frame "手柄开启力" {
                n290 = stacked-sequence {
                  frame #0 {
                    n291 = call "设备状态.vi"("枚举"=enum16{"Read", "Write"}."Write", "Status_Write"=i16 122 ("设备状态")) -> ()  [unwired: 9 in, 1 out]
                  }
                  frame #1 {
                    n292 = Wait (ms)(milliseconds to wait=u32 500 ("等待时间（毫秒）")) -> ()  [unwired: 1 out]
                  }
                  frame #2 {
                  }
                }
              }
              frame "手柄推拉力" {
                n293 = call "设备状态.vi"("枚举"=enum16{"Read", "Write"}."Write", "Status_Write"=i16 130 ("设备状态")) -> ()  [unwired: 9 in, 1 out]
              }
              frame "完成" {
                n294 = call "设备状态.vi"("枚举"=enum16{"Read", "Write"}."Write", "Status_Write"=i16 130 ("设备状态")) -> ()  [unwired: 9 in, 1 out]
              }
              frame "逆向空载" {
                n295 = call "设备状态.vi"("枚举"=enum16{"Read", "Write"}."Write", "Status_Write"=i16 152 ("设备状态")) -> ()  [unwired: 9 in, 1 out]
              }
              frame "手柄保持力" {
                n296 = call "设备状态.vi"("枚举"=enum16{"Read", "Write"}."Write", "Status_Write"=i16 130 ("设备状态")) -> ()  [unwired: 9 in, 1 out]
              }
            }
            n297 = local write "STEP"(w348) -> ()
          }
          frame "自动" {
            n298 = global read "Global.vi" "设备状态"() -> (w367:i16)
            n299 = case shown="1000" w367 {
              frame -128 {
                n300 = global write "Global.vi" "计时开始"(FALSE ("计时开始")) -> ()
                n301 = call "浮动通知.vi"("通知内容"="复位中……" ("Status")) -> ()  [unwired: 11 in]
              }
              frame 0 {
                n302 = global write "Global.vi" "计时开始"(FALSE ("计时开始")) -> ()
                n303 = call "浮动通知.vi"("通知内容"="手动状态！" ("Status")) -> ()  [unwired: 11 in]
              }
              frame 1 {
                n304 = call "浮动通知.vi"("通知内容"="请复位！" ("Status")) -> ()  [unwired: 11 in]
              }
              frame 4 {
                n305 = call "浮动通知.vi"("通知内容"="复位完成" ("Status")) -> ()  [unwired: 11 in]
                n306 = global write "Global.vi" "计时开始"(FALSE ("计时开始")) -> ()
              }
              frame 8 {
                n307 = call "浮动通知.vi"("通知内容"="程序停止！" ("Status")) -> ()  [unwired: 11 in]
              }
              frame 40 {
                n308 = call "曲线状态.vi"("枚举"=enum16{"Read", "Write"}."Read") -> ("Status_Read"=w377:i16)  [unwired: 10 in]
                n309 = case shown="2" w377 {
                  frame 0, Default {
                  }
                  frame 2 {
                    n310 = global read "A180648.vi" "手柄锁紧扭矩比例"() -> (w378:dbl)
                    n311 = call "传感器数据.vi"() -> ("电机角度"=w381:sgl, "扭矩"=w380:sgl)  [unwired: 6 in, 4 out]
                    n312 = local read "空载正向初始化"() -> (w387:bool)
                    n313 = Multiply(x=w380, y=w378) -> (x*y=w379:dbl)
                    n314 = local read "锁紧/开启初始化"() -> (w382:bool)
                    n315 = control-ref of="手柄锁紧力试验"() -> (w386:refnum<vi>)
                    n316 = call "曲线采集.vi"("曲线引用"=w386, "曲线索引"=0, "X"=w381, "Y"=w379) -> ("错误输出"=w384:errorcluster)  [unwired: 10 in, 1 out]
                    n317 = disable-structure shown="禁用" {
                      disable-tunnel: w387 -> [w393 _]
                      frame Disabled {
                        w392 = 2 ("Averaging Size")
                        n318 = call-poly <userlib>:"MGI Running Average.vi"("Averaging Size"=w392, "Initialize? (F)"=w393) -> ()  [unwired: 9 in, 1 out]
                        n319 = call-poly <userlib>:"MGI Running Average.vi"("Averaging Size"=w392, "Initialize? (F)"=w393) -> ()  [unwired: 9 in, 1 out]
                      }
                      frame Enabled {
                      }
                    }
                    n320 = Unbundle By Name(w384) -> ("status"=w383:bool)
                    n321 = local write "空载正向初始化"(w383) -> ()
                    n322 = case shown="真" w382 {
                      tunnel: w381 -> [_ w389]
                      tunnel: w379 -> [_ w388]
                      frame False {
                      }
                      frame True {
                        n323 = control-ref of="锁紧/开启"() -> (w390:refnum<vi>)
                        n324 = call "曲线采集.vi"("曲线引用"=w390, "曲线索引"=0, "X"=w389, "Y"=w388) -> ()  [unwired: 10 in, 2 out]
                      }
                    }
                  }
                }
              }
              frame 41 {
                n325 = local write "STEP"("判定" ("STEP")) -> ()
              }
              frame 50 {
                n326 = call "曲线状态.vi"("枚举"=enum16{"Read", "Write"}."Read") -> ("Status_Read"=w396:i16)  [unwired: 10 in]
                n327 = case shown="1" w396 {
                  frame 0, Default {
                  }
                  frame 1 {
                    n328 = global read "A180648.vi" "手柄开启扭矩比例"() -> (w397:dbl)
                    n329 = call "传感器数据.vi"() -> ("电机角度"=w401:sgl, "扭矩"=w400:sgl)  [unwired: 6 in, 4 out]
                    n330 = disable-structure shown="禁用" {
                      disable-tunnel: [w414 _] -> w406
                      disable-tunnel: [w413 _] -> _
                      frame Disabled {
                        w413 = 2 ("Averaging Size")
                        n331 = local read "功能逆向初始化"() -> (w414:bool)
                        n332 = call-poly <userlib>:"MGI Running Average.vi"("Averaging Size"=w413, "Initialize? (F)"=w414) -> ()  [unwired: 9 in, 1 out]
                        n333 = call-poly <userlib>:"MGI Running Average.vi"("Averaging Size"=w413, "Initialize? (F)"=w414) -> ()  [unwired: 9 in, 1 out]
                      }
                      frame Enabled {
                      }
                    }
                    n334 = Multiply(x=w400, y=w397) -> (x*y=w398:dbl)
                    n335 = control-ref of="手柄开启力试验"() -> (w404:refnum<vi>)
                    n336 = disable-structure shown="禁用" {
                      disable-tunnel: w406 -> [w412 _]
                      disable-tunnel: _ -> [w411 _]
                      frame Disabled {
                        n337 = call-poly <userlib>:"MGI Running Average.vi"("Averaging Size"=w411, "Initialize? (F)"=w412) -> ()  [unwired: 9 in, 1 out]
                      }
                      frame Enabled {
                      }
                    }
                    n338 = call "曲线采集.vi"("曲线引用"=w404, "曲线索引"=0, "X"=w401, "Y"=w398) -> ("错误输出"=w403:errorcluster)  [unwired: 10 in, 1 out]
                    n339 = Unbundle By Name(w403) -> ("status"=w402:bool)
                    n340 = local read "锁紧/开启初始化"() -> (w399:bool)
                    n341 = local write "功能逆向初始化"(w402) -> ()
                    n342 = case shown="真" w399 {
                      tunnel: w401 -> [_ w408]
                      tunnel: w398 -> [_ w407]
                      frame False {
                      }
                      frame True {
                        n343 = control-ref of="锁紧/开启"() -> (w410:refnum<vi>)
                        n344 = call "曲线采集.vi"("曲线引用"=w410, "曲线索引"=1, "X"=w408, "Y"=w407) -> ()  [unwired: 10 in, 2 out]
                      }
                    }
                  }
                }
              }
              frame 51 {
                n345 = global write "Global.vi" "STOP_NVH"(TRUE ("STOP_NVH")) -> ()
                n346 = local write "STEP"("判定" ("STEP")) -> ()
              }
              frame 52 {
                n347 = call "浮动通知.vi"("通知内容"="手柄力不合格请调整！") -> ()  [unwired: 11 in]
              }
              frame 54 {
                n348 = call "浮动通知.vi"("通知内容"="调整后请点击触摸屏按钮继续") -> ()  [unwired: 11 in]
              }
              frame 60 {
                n349 = call "曲线状态.vi"("枚举"=enum16{"Read", "Write"}."Read") -> ("Status_Read"=w420:i16)  [unwired: 10 in]
                n350 = case shown="3" w420 {
                  frame 0, Default {
                  }
                  frame 3 {
                    n351 = disable-structure shown="禁用" {
                      frame Disabled {
                        w431 = 2 ("Averaging Size")
                        n352 = local read "空载逆向初始化"() -> (w432:bool)
                        n353 = call-poly <userlib>:"MGI Running Average.vi"("Averaging Size"=w431, "Initialize? (F)"=w432) -> ()  [unwired: 9 in, 1 out]
                        n354 = call-poly <userlib>:"MGI Running Average.vi"("Averaging Size"=w431, "Initialize? (F)"=w432) -> ()  [unwired: 9 in, 1 out]
                      }
                      frame Enabled {
                      }
                    }
                    n355 = call "传感器数据.vi"() -> ("拉压力"=w425:sgl, "电缸位移"=w426:sgl)  [unwired: 6 in, 4 out]
                    n356 = global read "A180648.vi" "管柱推拉力比例"() -> (w421:dbl)
                    n357 = control-ref of="角度调节力试验"() -> (w430:refnum<vi>)
                    n358 = Multiply(x=sgl 1000.0, y=w425) -> (x*y=w424:sgl)
                    n359 = Multiply(x=w421, y=w424) -> (x*y=w422:dbl)
                    n360 = call "曲线采集.vi"("曲线引用"=w430, "曲线索引"=0, "X"=w426, "Y"=w422) -> ("错误输出"=w428:errorcluster)  [unwired: 10 in, 1 out]
                    n361 = Unbundle By Name(w428) -> ("status"=w427:bool)
                    n362 = local write "空载逆向初始化"(w427) -> ()
                  }
                }
              }
              frame 61 {
                n363 = local write "STEP"("判定" ("STEP")) -> ()
              }
              frame 70 {
                n364 = call "曲线状态.vi"() -> ("Status_Read"=w434:i16)  [unwired: 11 in]
                n365 = case shown="4" w434 {
                  frame 0, Default {
                  }
                  frame 4 {
                    n366 = control-ref of="管柱保持力试验"() -> (w440:refnum<vi>)
                    n367 = call "传感器数据.vi"() -> ("拉压力"=w435:sgl, "电缸位移"=w438:sgl)  [unwired: 6 in, 4 out]
                    n368 = Multiply(x=sgl 1000.0, y=w435) -> (x*y=w437:sgl)
                    n369 = call "曲线采集.vi"("曲线引用"=w440, "曲线索引"=0, "X"=w438, "Y"=w437) -> ()  [unwired: 10 in, 2 out]
                  }
                }
              }
              frame 71 {
                n370 = local write "STEP"("判定" ("STEP")) -> ()
              }
              frame 100 {
                n371 = call "浮动通知.vi"("通知内容"="请放入产品后按启动按钮！" ("Status")) -> ()  [unwired: 11 in]
              }
              frame 101 {
                n372 = local write "STEP"("扫码" ("STEP")) -> ()
              }
              frame 113 {
                n373 = call "设备状态.vi"("枚举"=enum16{"Read", "Write"}."Write", "Status_Write"=i16 114 ("设备状态")) -> ()  [unwired: 9 in, 1 out]
                n374 = local write "STEP"("等待" ("STEP")) -> ()
              }
              frame 999 {
                n375 = call "浮动通知.vi"("通知内容"="请启动！" ("Status")) -> ()  [unwired: 11 in]
              }
              frame 1000 {
                n376 = local write "STEP"("初始化" ("STEP")) -> ()
              }
              frame 1024 {
                n377 = local write "STEP"("退出自动" ("STEP")) -> ()
              }
              frame Default {
              }
            }
          }
          frame "合格判定" {
            n378 = Wait (ms)(milliseconds to wait=u32 100 ("等待时间（毫秒）")) -> ()  [unwired: 1 out]
            n379 = local write "STEP"("等待" ("STEP")) -> ()
          }
          frame "报表" {
            n380 = stacked-sequence {
              seq-local: [_ w458 _ _] -> [_ _ w462 _]
              frame #0 {
                n381 = global write "Global.vi" "计时开始"(FALSE ("计时开始")) -> ()
              }
              frame #1 {
                n382 = Wait (ms)(milliseconds to wait=u32 100 ("等待时间（毫秒）")) -> ()  [unwired: 1 out]
                n383 = global read "Global.vi" "产品编号"() -> (w454:string)
                n384 = call <vilib>:"Space Constant.vi"() -> ("String"=w455:string)
                n385 = call "时间秒.vi"() -> ("结果字符串"=w456:string)  [unwired: 11 in]
                n386 = Concatenate Strings(w454, w455, w456) -> (w453:string)
                n387 = call "Report.vi"("文件重命名"=TRUE, "文件名称"=w453, "检测结果"="判定结果") -> ("PRODUCT_VAULE"=w458:string)  [unwired: 7 in, 1 out]
              }
              frame #2 {
                n388 = global read "Global.vi" "联机模式"() -> (w461:enum16{"单机", "追溯"})
                n389 = case shown="\"追溯\"" w461 {
                  tunnel: w462 -> [_ w463]
                  frame "单机", Default {
                  }
                  frame "追溯" {
                    n390 = global read "Global.vi" "Result"() -> (w465:refnum<vi>)
                    n391 = property class="Tbl"(reference=w465) -> (reference out=w470:refnum<vi>, error out=w467:errorcluster, "Row Headers[]"=w468:string[])  [unwired: 1 in]
                    n392 = property class="Tbl"(reference=w470, error in=w467) -> (error out=w466:errorcluster, "Value"=w469:string[][])  [unwired: 1 out]
                    n393 = for {
                      tunnel: w469 -> [w477] mode=indexing
                      tunnel: w468 -> [w478] mode=indexing
                      tunnel: [w475] -> w464 mode=indexing if=w476
                      shift-right: [w474] -> _
                      shift-left: w466 -> [w474]
                      n394 = Build Array (concatenate)(w478, w477) -> (w475:string[])
                      n395 = Index Array(array=w477) -> (element=w479:string)  [unwired: 1 in]
                      n396 = case shown="默认" w479 {
                        tunnel: [TRUE FALSE] -> w476
                        frame Default {
                        }
                        frame "" {
                        }
                      }
                    }
                    n397 = global read "追溯Global.vi" "DEVICE_ID"() -> (w472:string)
                    n398 = global read "追溯Global.vi" "CODE_ID"() -> (w473:string)
                    n399 = global read "追溯Global.vi" "USER_ID"() -> (w471:string)
                    n400 = call "UPTEST.vi"("Result"=w464, "CODE_ID"=w473, "DEVICE_ID"=w472) -> ()  [unwired: 6 in, 1 out]
                    n401 = call "UPRESULT.vi"("DEVICE_ID"=w472, "USER_ID"=w471, "CODE_ID"=w473, "RESULT_VALUE"=w463) -> ()  [unwired: 11 in, 1 out]
                  }
                }
              }
              frame #3 {
                n402 = local write "STEP"("进入自动" ("STEP")) -> ()
              }
            }
          }
        }
        n403 = global read "Global.vi" "程序关闭"() -> (w21:bool)
      }
      n404 = while {
        shift-right: [w484] -> w19
        shift-left: w18 -> [w485]
        stop <- w486 stop-if-true
        n405 = event shown="[0] 超时" {
          selector: w485 -> [_ _ _ _ _ _ _ _ _]
          dyn-events: [_ _ _ _ _ _ _ _ _] -> w484
          timeout: 200 -> [_ _ _ _ _ _ _ _ _]
          event Timeout {
            n406 = event-data() -> ()  [unwired: 1 in, 3 out]
            n407 = call "Obtain Broadcast Events for Registration.vi"() -> ("Already running?"=w488:bool)  [unwired: 9 in, 2 out]
            n408 = case shown="真" w488 {
              frame False {
                n409 = local write "STEP"("手动" ("STEP")) -> ()
              }
              frame True {
                n410 = call "错误代码.vi"() -> ("Status_Read"=w490:u32)  [unwired: 11 in]
                n411 = feedback #1() -> (w500:u32)  [unwired: 1 in]
                n412 = feedback-in #1(w490) -> ()
                n413 = case shown="0" w490 {
                  frame 0 {
                    n414 = global read "Global.vi" "报警图标"() -> (w501:refnum<vi>)
                    n415 = property class="Bool"(reference=w501, "Visible"=FALSE ("可见")) -> ()  [unwired: 1 in, 2 out]
                  }
                  frame 1, Default {
                    n416 = global read "Global.vi" "报警图标"() -> (w504:refnum<vi>)
                    n417 = property class="Bool"(reference=w504, "Visible"=TRUE ("可见")) -> ()  [unwired: 1 in, 2 out]
                  }
                }
                n418 = Greater Or Equal?(x=w490, y=i16 5000) -> (x >= y?=w498:bool)
                n419 = Less?(x=w490, y=i16 5200) -> (x < y?=w499:bool)
                n420 = Equal?(x=w490, y=w500) -> (x = y?=w497:bool)
                n421 = global read "Global.vi" "报警图标"() -> (w492:refnum<vi>)
                n422 = And(x=w498, y=w499) -> (x .and. y?=w491:bool)
                n423 = property class="Bool"(reference=w492, "Value"=w491) -> ()  [unwired: 1 in, 2 out]
                n424 = Bundle By Name(cluster=errorcluster {"status"=FALSE, "code"=0, "source"=""} ("错误常量"), "status"=w491, "code"=w490) -> (w496:errorcluster)
                n425 = case shown="假" w497 {
                  tunnel: w496 -> [w505 _]
                  frame False {
                    n426 = call "报警处理.vi"("错误常量"=w505) -> ()  [unwired: 9 in, 2 out]
                  }
                  frame True {
                  }
                }
              }
            }
          }
          event User Event {
            n427 = event-data() -> ("产品标尺"=w506:string)  [unwired: 1 in, 4 out]
            n428 = control-ref of="管柱保持力试验"() -> (w511:refnum<vi>)
            n429 = control-ref of="手柄锁紧力试验"() -> (w507:refnum<vi>)
            n430 = control-ref of="锁紧/开启"() -> (w510:refnum<vi>)
            n431 = control-ref of="手柄开启力试验"() -> (w509:refnum<vi>)
            n432 = control-ref of="角度调节力试验"() -> (w512:refnum<vi>)
            n433 = Build Array(w511, w509, w510, w512, w507) -> (w508:refnum<vi>[])
            n434 = for {
              tunnel: w508 -> [w514] mode=indexing
              tunnel: w506 -> [w513]
              n435 = call "XY_conf.vi"("方式"=enum16{"写入", "读取"}."读取", "产品"=w513, "XY图引用"=w514) -> ()  [unwired: 4 in, 1 out]
            }
          }
          event User Event {
            n436 = event-data() -> ("试验项"=→"试验项目":T1)  [unwired: 1 in]
            n437 = disable-structure shown="禁用" {
              frame Disabled {
                n438 = local read "管柱保持力试验"() -> (w520:cluster{dbl[], dbl[]}[])
                n439 = global read "判定参数.vi" "最大位移"() -> (w517:dbl)
                n440 = global read "判定参数.vi" "最大拉力"() -> (w519:dbl)
                n441 = global read "判定参数.vi" "最小拉力"() -> (w518:dbl)
                n442 = for {
                  tunnel: [w527] -> w521 mode=indexing
                  tunnel: w520 -> [w526] mode=indexing
                  tunnel: w519 -> [w525]
                  tunnel: w518 -> [w524]
                  tunnel: w517 -> [w523]
                  tunnel: w517 -> [w522]
                  i -> [w528]
                  n443 = case shown="1" w528 {
                    tunnel: [w529 w530] -> w527
                    tunnel: w526 -> [w529 _]
                    tunnel: w525 -> [_ w534]
                    tunnel: w524 -> [_ w533]
                    tunnel: w523 -> [_ w532]
                    tunnel: w522 -> [_ w531]
                    frame 0, Default {
                    }
                    frame 1 {
                      n444 = Build Array(w532, w532, w531, w531, w532) -> (w536:dbl[])
                      n445 = Build Array(w533, w534, w534, w533, w533) -> (w535:dbl[])
                      n446 = Bundle(w536, w535) -> (w530:cluster{dbl[], dbl[]})  [unwired: 1 in]
                    }
                  }
                }
                n447 = local write "管柱保持力试验"(w521) -> ()
              }
              frame Enabled {
              }
            }
            n448 = disable-structure shown="禁用" {
              disable-tunnel: _ -> [w537 _]
              frame Disabled {
                n449 = global read "A180648.vi" "检测结果"() -> (w540:string[][][])
                n450 = global read "Global.vi" "Result"() -> (w538:refnum<vi>)
                n451 = Index Array(array=w540, index (dim 0)=w537) -> (element=w539:string[][])  [unwired: 2 in]
                n452 = property class="Tbl"(reference=w538, "Value"=w539) -> ()  [unwired: 1 in, 2 out]
              }
              frame Enabled {
              }
            }
          }
          event "试验项目": Value Change {
            n453 = event-data() -> ("NewVal"=w541:T1)  [unwired: 1 in]
            n454 = disable-structure shown="禁用" {
              disable-tunnel: w541 -> [w545 _]
              frame Disabled {
                n455 = global read "A180648.vi" "检测结果"() -> (w544:string[][][])
                n456 = global read "Global.vi" "Result"() -> (w542:refnum<vi>)
                n457 = Index Array(array=w544, index (dim 0)=w545) -> (element=w543:string[][])  [unwired: 2 in]
                n458 = property class="Tbl"(reference=w542, "Value"=w543) -> ()  [unwired: 1 in, 2 out]
              }
              frame Enabled {
              }
            }
          }
          event "管柱保持力试验", "锁紧/开启", "角度调节力试验", "手柄锁紧力试验", "手柄开启力试验", "逆向空载试验": Scale Range Change {
            n459 = event-data() -> ("CtlRef"=w548:refnum<vi>)  [unwired: 1 in, 4 out]
            n460 = global read "Global.vi" "产品型号"() -> (w546:string)
            n461 = call "XY_conf.vi"("方式"=enum16{"写入", "读取"}."写入", "产品"=w546, "XY图引用"=w548) -> ()  [unwired: 4 in, 1 out]
          }
          event Panel Close {
            n462 = event-data() -> ()  [unwired: 1 in, 4 out]
            n463 = global write "Global.vi" "程序关闭"(TRUE ("程序关闭")) -> ()
          }
          event "管柱保持力试验", "锁紧/开启", "角度调节力试验", "振动1NVH-FFT", "手柄锁紧力试验", "手柄开启力试验", "逆向空载试验": Mouse Enter; "管柱保持力试验", "锁紧/开启", "角度调节力试验", "振动1NVH-FFT", "手柄锁紧力试验", "手柄开启力试验", "逆向空载试验": Mouse Leave; "管柱保持力试验", "锁紧/开启", "角度调节力试验", "振动1NVH-FFT", "手柄锁紧力试验", "手柄开启力试验", "逆向空载试验": Cursor Move {
            n464 = event-data() -> ("CtlRef"=w552:refnum<vi>, "Type"=w550:T9)  [unwired: 1 in]
            n465 = call "CursorShow.vi"("nameShow"=TRUE, "Type"=w550, "Graph"=w552) -> ()  [unwired: 7 in, 2 out]
          }
          event "管柱保持力试验", "锁紧/开启", "角度调节力试验", "振动1NVH-FFT", "手柄锁紧力试验", "手柄开启力试验", "逆向空载试验": Mouse Down {
            n466 = event-data() -> ("CtlRef"=w557:refnum<vi>, "Coords"=w556:T10, "Type"=w554:T9)  [unwired: 1 in]
            n467 = invoke class="WFGraph" method="Map Coords To XY"(reference=w557, "Coords"=w556) -> (reference out=w555:refnum<vi>, "XY"=w553:cluster{"X":dbl, "Y":dbl})  [unwired: 5 in, 5 out]
            n468 = call "CursorShow.vi"("游标.游标位置"=w553, "Type"=w554, "Graph"=w555) -> ()  [unwired: 7 in, 2 out]
          }
          event "更换坐标": Value Change {
            w572 = 1 ("索引")
            w573 = 1 ("索引")
            w587 = 1 ("索引")
            n469 = event-data() -> ()  [unwired: 1 in, 5 out]
            n470 = global read "A180648.vi" "坐标参数"() -> (w605:string[][])
            n471 = Index Array(array=w605) -> (element #1=w604:string[], element #2=w597:string[], element #3=w592:string[], element #4=w586:string[])  [unwired: 8 in]
            n472 = Index Array(array=w604, index #1=1 ("索引")) -> (element #1=w603:string, element #2=w600:string)  [unwired: 1 in]
            n473 = Index Array(array=w592, index #1=w587) -> (element #1=w591:string, element #2=w590:string)  [unwired: 1 in]
            n474 = Index Array(array=w586, index #1=w587) -> (element #1=w588:string, element #2=w589:string)  [unwired: 1 in]
            n475 = Index Array(array=w597, index #1=1 ("索引")) -> (element #1=w596:string, element #2=w595:string)  [unwired: 1 in]
            n476 = Fract/Exp String To Number(string=w603) -> (number=w602:dbl)  [unwired: 3 in, 1 out]
            n477 = Fract/Exp String To Number(string=w600) -> (number=w601:dbl)  [unwired: 3 in, 1 out]
            n478 = Fract/Exp String To Number(string=w596) -> (number=w594:dbl)  [unwired: 3 in, 1 out]
            n479 = Fract/Exp String To Number(string=w595) -> (number=w593:dbl)  [unwired: 3 in, 1 out]
            n480 = Fract/Exp String To Number(string=w590) -> (number=w584:dbl)  [unwired: 3 in, 1 out]
            n481 = Fract/Exp String To Number(string=w591) -> (number=w585:dbl)  [unwired: 3 in, 1 out]
            n482 = Fract/Exp String To Number(string=w589) -> (number=w582:dbl)  [unwired: 3 in, 1 out]
            n483 = Fract/Exp String To Number(string=w588) -> (number=w583:dbl)  [unwired: 3 in, 1 out]
            n484 = property on="手柄锁紧力试验" class="XYGraph (严格)"("XScale.Minimum"=w602) -> ()  [unwired: 2 in, 2 out]
            n485 = property on="手柄锁紧力试验" class="XYGraph (严格)"("XScale.Maximum"=w601) -> ()  [unwired: 2 in, 2 out]
            n486 = property on="手柄锁紧力试验" class="XYGraph (严格)"("YScale.Minimum"=w594) -> ()  [unwired: 2 in, 2 out]
            n487 = property on="手柄锁紧力试验" class="XYGraph (严格)"("YScale.Maximum"=w593) -> ()  [unwired: 2 in, 2 out]
            n488 = property on="手柄开启力试验" class="XYGraph (严格)"("XScale.Minimum"=w585) -> ()  [unwired: 2 in, 2 out]
            n489 = property on="手柄开启力试验" class="XYGraph (严格)"("XScale.Maximum"=w584) -> ()  [unwired: 2 in, 2 out]
            n490 = property on="手柄开启力试验" class="XYGraph (严格)"("YScale.Maximum"=w582) -> ()  [unwired: 2 in, 2 out]
            n491 = property on="手柄开启力试验" class="XYGraph (严格)"("YScale.Minimum"=w583) -> ()  [unwired: 2 in, 2 out]
            n492 = global read "A180648.vi" "坐标参数"() -> (w581:string[][])
            n493 = Index Array(array=w581, index (row) #1=4 ("索引 (行)")) -> (element #1=w575:string[], element #2=w574:string[], element #3=w567:string[], element #4=w566:string[])  [unwired: 7 in]
            n494 = Index Array(array=w575, index #1=w573) -> (element #1=w576:string, element #2=w577:string)  [unwired: 1 in]
            n495 = Index Array(array=w574, index #1=w573) -> (element #1=w579:string, element #2=w578:string)  [unwired: 1 in]
            n496 = Index Array(array=w567, index #1=w572) -> (element #1=w571:string, element #2=w570:string)  [unwired: 1 in]
            n497 = Index Array(array=w566, index #1=w572) -> (element #1=w568:string, element #2=w569:string)  [unwired: 1 in]
            n498 = Fract/Exp String To Number(string=w577) -> (number=w564:dbl)  [unwired: 3 in, 1 out]
            n499 = Fract/Exp String To Number(string=w576) -> (number=w565:dbl)  [unwired: 3 in, 1 out]
            n500 = Fract/Exp String To Number(string=w578) -> (number=w562:dbl)  [unwired: 3 in, 1 out]
            n501 = Fract/Exp String To Number(string=w579) -> (number=w563:dbl)  [unwired: 3 in, 1 out]
            n502 = Fract/Exp String To Number(string=w570) -> (number=w560:dbl)  [unwired: 3 in, 1 out]
            n503 = Fract/Exp String To Number(string=w571) -> (number=w561:dbl)  [unwired: 3 in, 1 out]
            n504 = Fract/Exp String To Number(string=w569) -> (number=w558:dbl)  [unwired: 3 in, 1 out]
            n505 = Fract/Exp String To Number(string=w568) -> (number=w559:dbl)  [unwired: 3 in, 1 out]
            n506 = property on="角度调节力试验" class="XYGraph (严格)"("XScale.Minimum"=w565) -> ()  [unwired: 2 in, 2 out]
            n507 = property on="角度调节力试验" class="XYGraph (严格)"("XScale.Maximum"=w564) -> ()  [unwired: 2 in, 2 out]
            n508 = property on="角度调节力试验" class="XYGraph (严格)"("YScale.Minimum"=w563) -> ()  [unwired: 2 in, 2 out]
            n509 = property on="角度调节力试验" class="XYGraph (严格)"("YScale.Maximum"=w562) -> ()  [unwired: 2 in, 2 out]
            n510 = property on="管柱保持力试验" class="XYGraph (严格)"("XScale.Minimum"=w561) -> ()  [unwired: 2 in, 2 out]
            n511 = property on="管柱保持力试验" class="XYGraph (严格)"("XScale.Maximum"=w560) -> ()  [unwired: 2 in, 2 out]
            n512 = property on="管柱保持力试验" class="XYGraph (严格)"("YScale.Minimum"=w559) -> ()  [unwired: 2 in, 2 out]
            n513 = property on="管柱保持力试验" class="XYGraph (严格)"("YScale.Maximum"=w558) -> ()  [unwired: 2 in, 2 out]
          }
        }
        n514 = control-ref of="更换坐标"() -> (w483:refnum<vi>)
        n515 = global write "Global.vi" "更换坐标"(w483) -> ()
        n516 = global read "Global.vi" "程序关闭"() -> (w486:bool)
      }
    }
  }
  n517 = Unregister For Events(event registration refnum=w6) -> ()  [unwired: 1 in, 1 out]
